vi "Load setting from file.vi"(8 "error in (no error)":errorcluster, 10 "settings path":string, 11 "ServiceManager in":refnum<class "ServiceManager.lvclass">) -> (0 "error out":errorcluster, 3 "ServiceManager out":refnum<class "ServiceManager.lvclass">)   [LabVIEW 2012, in "ServiceManager.lvclass"]
uses:
  ServiceManager.lvclass
  Murmex/LabVIEW/Murmex/ResetMessage/ResetMessage.lvclass
  settings_cluster.ctl
  Murmex/LabVIEW/Murmex/Murmex/component_specification_cluster.ctl
  ServiceManager.lvclass/ServiceManager.ctl
  Murmex/LabVIEW/Murmex/Murmex/Murmex.lvclass
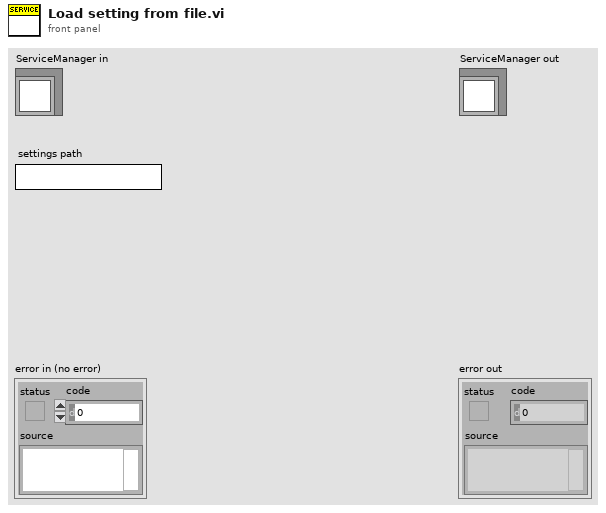
[diagram p1: front panel]
types:
  T1 = enum16{"open", "replace", "create", "open or create", "replace or create", "replace or create with confirmation"}
  T2 = typedef "ServiceManager.lvclass/settings_cluster.ctl" = cluster{"components":T3[]}
  T3 = typedef "Murmex.lvlib/Murmex.lvclass/component_specification_cluster.ctl" = cluster{"name":string, "language":string, "host name":string, "id":string}
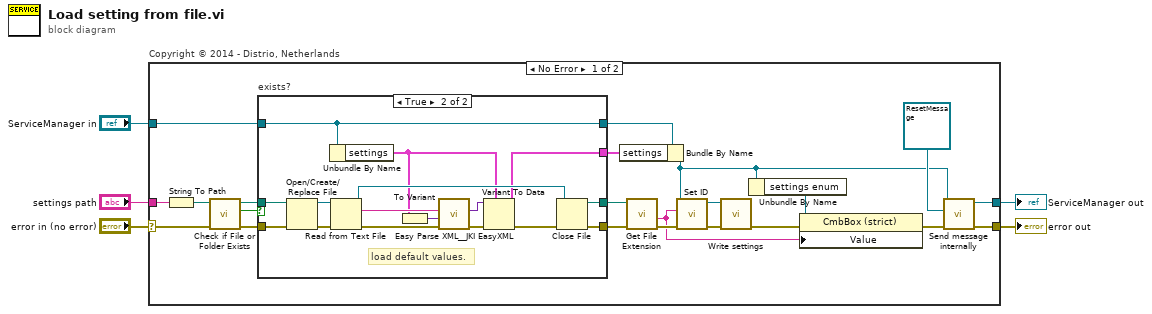
[diagram p0: block diagram]
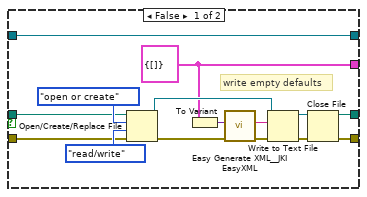
[diagram p2: hidden frame]
diagram:
  n1 = case "Copyright © 2014 - Distrio, Netherlands" shown="No Error" "error in (no error)" {
    selector: "error in (no error)" -> [w11 w60]
    tunnel: [w24 w60] -> w4
    tunnel: [w23 w59] -> w2
    tunnel: "ServiceManager in" -> [w10 w59]
    tunnel: "settings path" -> [w27 _]
    frame No Error {
      n2 = String To Path(string=w27) -> (path=w12:path)
      n3 = call <vilib>:"Check if File or Folder Exists.vi"("error in (no error)"=w11, "path"=w12) -> ("error out"=w13:errorcluster, "file or folder exists?"=w16:bool, "dup path"=w14:path)  [unwired: 7 in]
      n4 = case "exists?" shown="True" w16 {
        tunnel: w14 -> [w40 w54]
        tunnel: w13 -> [w39 w55]
        tunnel: [w32 w47] -> w7
        tunnel: [w29 w45] -> w15
        tunnel: w10 -> [w30 w44]
        tunnel: [w30 w44] -> w9
        tunnel: [w28 w43] -> w8
        frame False {
          w29 = T2 {"components"=[]} ("settings")
          # "write empty defaults"
          n5 = Open/Create/Replace File(file path (use dialog)=w40, error in=w39, operation (0:open)=T1."open or create", access (0:read/write)=enum16{"read/write", "read-only", "write-only"}."read/write") -> (refnum out=w34:refnum<file>, error out=w38:errorcluster)  [unwired: 2 in, 1 out]
          n6 = To Variant(anything=w29) -> (Variant=w31:variant)
          n7 = call <vilib>:"Easy Generate XML__JKI EasyXML.vi"("error in (no error)"=w38, "LabVIEW Data"=w31) -> ("error out"=w36:errorcluster, "XML String"=w37:string)  [unwired: 8 in]
          n8 = Write to Text File(file (use dialog)=w34, text=w37, error in=w36) -> (refnum out=w33:refnum<file>, error out=w35:errorcluster)  [unwired: 1 in, 1 out]
          n9 = Close File(refnum=w33, error in=w35) -> (path=w28:path, error out=w32:errorcluster)
        }
        frame True {
          # "load default values."
          n10 = Open/Create/Replace File(file path (use dialog)=w54, error in=w55) -> (refnum out=w52:refnum<file>, error out=w53:errorcluster)  [unwired: 4 in, 1 out]
          n11 = Unbundle By Name(w44) -> ("settings"=w46:T2)
          n12 = Read from Text File(file (use dialog)=w52, error in=w53) -> (refnum out=w49:refnum<file>, text=w51:string, error out=w50:errorcluster)  [unwired: 2 in, 1 out]
          n13 = To Variant(anything=w46) -> (Variant=w57:variant)
          n14 = call <vilib>:"Easy Parse XML__JKI EasyXML.vi"("error in (no error)"=w50, "LabVIEW Data (Type)"=w57, "XML String"=w51) -> ("error out"=w56:errorcluster, "LabVIEW Data"=w58:variant)  [unwired: 7 in]
          n15 = Variant To Data(error in=w56, type=w46, Variant=w58) -> (data=w45:T2, error out=w48:errorcluster)
          n16 = Close File(refnum=w49, error in=w48) -> (path=w43:path, error out=w47:errorcluster)
        }
      }
      n17 = Bundle By Name(cluster=w9, "settings"=w15) -> (w6:refnum<class "ServiceManager.lvclass">)
      n18 = call <vilib>:"Get File Extension.vi"("error in (no error)"=w7, "file"=w8) -> ("error out"=w26:errorcluster, "filename without extension"=w18:string)  [unwired: 6 in, 2 out]
      n19 = call "Set ID.vi"("error in (no error)"=w26, "id"=w18, "Murmex in"=w6) -> ("error out"=w19:errorcluster, "Murmex out"=w20:refnum<class "ServiceManager.lvclass">)  [unwired: 7 in]
      n20 = call-dynamic "Write settings.vi"("error in (no error)"=w19, "ServiceManager in"=w20) -> ("error out"=w17:errorcluster)  [unwired: 6 in, 3 out]
      n21 = Unbundle By Name(w6) -> ("settings enum"=w25:refnum<vi>)
      n22 = property class="CmbBox (strict)"(reference=w25, error in=w17, "Value"=w18) -> (error out=w21:errorcluster)  [unwired: 1 out]
      n23 = call "Send message internally.vi"("error in (no error)"=w21, "Message"=refnum<class "ResetMessage.lvclass"> refnum ("ResetMessage.lvclass"), "Murmex in"=w6) -> ("error out"=w24:errorcluster, "Murmex out"=w23:refnum<class "ServiceManager.lvclass">)  [unwired: 7 in]
    }
    frame Error {
    }
  }
  "error out" <- w4
  "ServiceManager out" <- w2
